vi "Agilent 33120A.vi"() -> ()   [LabVIEW 2018, in "com.Instrument.lvlib"]
doc: "Shows how to generate a standard waveform."
uses:
  com.Instrument.lvlib
  <instrlib>/Agilent 33XXX Series/Agilent 33XXX Series.lvlib
  Global.vi
panel:
  in  "Serial Configuration":T1={"Baud Rate"=9600, "Parity"=0, "Data Bits"=8, "Flow Control"=4} {"Flow Control" items=["None", "XON/XOFF", "RTS/CTS", "XON/XOFF & RTS/CTS", "DTR/DSR", "XON/XOFF & DTR/DSR"]; "Data Bits" items=["7"=7, "8"=8]; "Parity" items=["None", "Odd", "Even", "Mark", "Space"]; "Baud Rate" items=["300"=300, "600"=600, "1200"=1200, "2400"=2400, "4800"=4800, "9600"=9600, "19200"=19200]}
  in  "VISA resource name":refnum<visa-resource-name>
  # "(c) 2005 - 2013 National Instruments.  ALL RIGHTS RESERVED."
  # "According to the project specification,\nall parameters are set to constant.\nFrequency: 20Hz\nWaveform Function: Triangle\nAmplitude: 10 Vpp\nDC Offset: 0V\nUnit: Vpp"
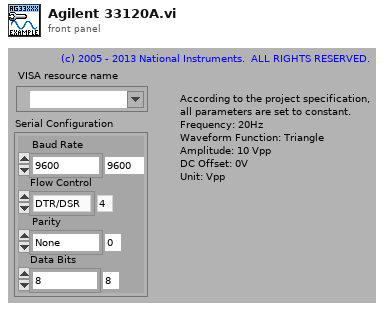
[diagram p1: front panel]
types:
  T1 = cluster{"Baud Rate":u32, "Parity":u16, "Data Bits":u16, "Flow Control":u16}
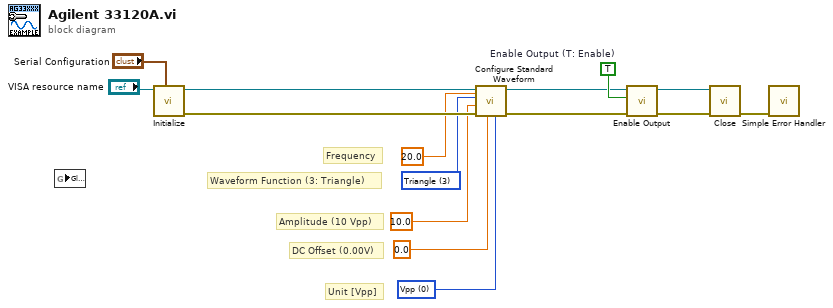
[diagram p0: block diagram]
diagram:
  w2 = u16 0 items=["Vpp", "Vrms", "dB"] ("Unit (0: Vpp)")
  w4 = u16 3 items=["DC", "Sine", "Square", "Triangle", "Ramp", "Pulse", "Noise", "Sinc", "Negative Ramp", "Exponential Rise", "Exponential Fall", "Cardiac"] ("Waveform Function (1: Sine)")
  w10 = TRUE  # Enable Output (T: Enable)
  # "Unit [Vpp]"
  # "DC Offset (0.00V)"
  # "Amplitude (10 Vpp)"
  # "Waveform Function (3: Triangle)"
  # "Frequency"
  n1 = global read "Global.vi" item#-1() -> ()  [unwired: 1 in]
  n2 = call <instrlib>:"Initialize.vi"("Serial Configuration"="Serial Configuration", "VISA resource name"="VISA resource name") -> ("error out"=w13:errorcluster, "VISA resource name out"=w14:refnum<visa-resource-name>)  [unwired: 8 in]
  n3 = call <instrlib>:"Configure Standard Waveform.vi"("Unit (0: Vpp)"=w2, "DC Offset (0.00 V)"=0.0, "Frequency (1000 Hz)"=20.0, "error in (no error)"=w13, "Amplitude (1)"=10.0, "Waveform Function (1: Sine)"=w4, "VISA resource name"=w14) -> ("error out"=w8:errorcluster, "VISA resource name out"=w9:refnum<visa-resource-name>)  [unwired: 3 in]
  n4 = call <instrlib>:"Enable Output.vi"("error in (no error)"=w8, "Enable Output  (T: Enable)"=w10, "VISA resource name"=w9) -> ("error out"=w6:errorcluster, "VISA resource name out"=w7:refnum<visa-resource-name>)  [unwired: 7 in]
  n5 = call <instrlib>:"Close.vi"("error in (no error)"=w6, "VISA resource name"=w7) -> ("error out"=w12:errorcluster)  [unwired: 9 in]
  n6 = call <vilib>:"Simple Error Handler.vi"("error in (no error)"=w12) -> ()  [unwired: 4 in, 5 out]
